vi "LVIS_SendToLog.vi"(8 "Error In":errorcluster, 11 "EventData":string) -> (0 "Error Out":errorcluster)   [LabVIEW 2015]
doc: "If enabled in the LVIS_Settings file, sends event data to the event log."
uses:
  Globals/LVIS_DcGlobals.vi
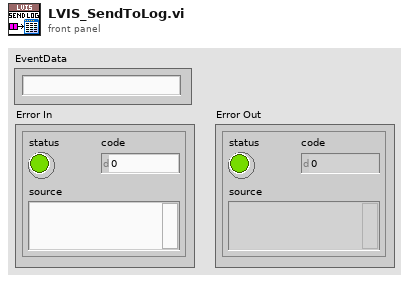
[diagram p1: front panel]
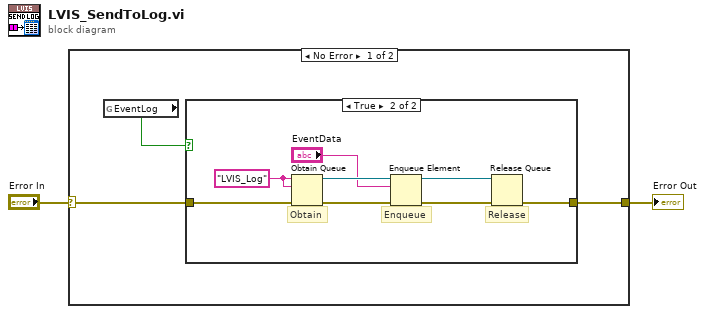
[diagram p0: block diagram]
diagram:
  n1 = case shown="No Error" "Error In" {
    selector: "Error In" -> [w5 w15]
    tunnel: [w4 w15] -> w1
    frame No Error {
      n2 = global read "LVIS_DcGlobals.vi" "EventLog"() -> (w3:bool)
      n3 = case shown="True" w3 {
        tunnel: w5 -> [w6 w14]
        tunnel: [w6 w7] -> w4
        frame False {
          # "Event logging is disabled"
        }
        frame True {
          w13 = "LVIS_Log" ("name (unnamed)")
          # "Release"
          # "Enqueue"
          # "Obtain"
          n4 = Obtain Queue(name (unnamed)=w13, element data type=w13, error in (no error)=w14) -> (queue out=w11:refnum<queue>, error out=w12:errorcluster)  [unwired: 2 in, 1 out]
          n5 = Enqueue Element(queue=w11, element="EventData", error in (no error)=w12) -> (queue out=w8:refnum<queue>, error out=w9:errorcluster)  [unwired: 1 in, 1 out]
          n6 = Release Queue(queue=w8, error in (no error)=w9) -> (error out=w7:errorcluster)  [unwired: 1 in, 2 out]
        }
      }
    }
    frame Error {
    }
  }
  "Error Out" <- w1
